vi "Calculate Center.vi"(8 "Type of Assembly Tray":i32, 9 "Syringe Coordinates":dbl[](array[numeric]), 10 "Relative Coordinates":dbl[][](array[numeric]), 11 "Fiducial Measurements":dbl[][](array[numeric])) -> (3 "XYZTheta Centers":dbl[][](array[numeric]))   [LabVIEW 2019, in "Assembly Tray.lvclass"]
uses:
  Assembly Tray.lvclass
  <vilib>/Analysis/coordinate.llb/2D Cartesian Coordinate Rotation (Scalar).vi
  <vilib>/Analysis/NI_AALPro.lvlib
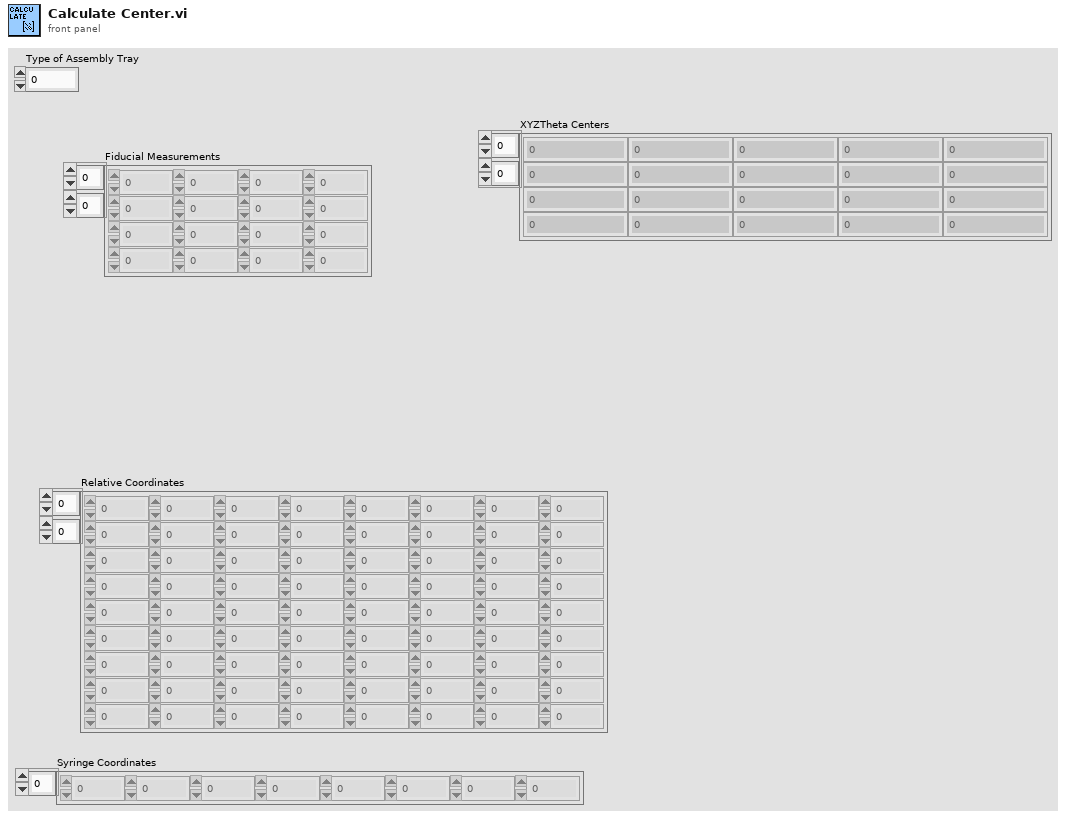
[diagram p1: front panel]
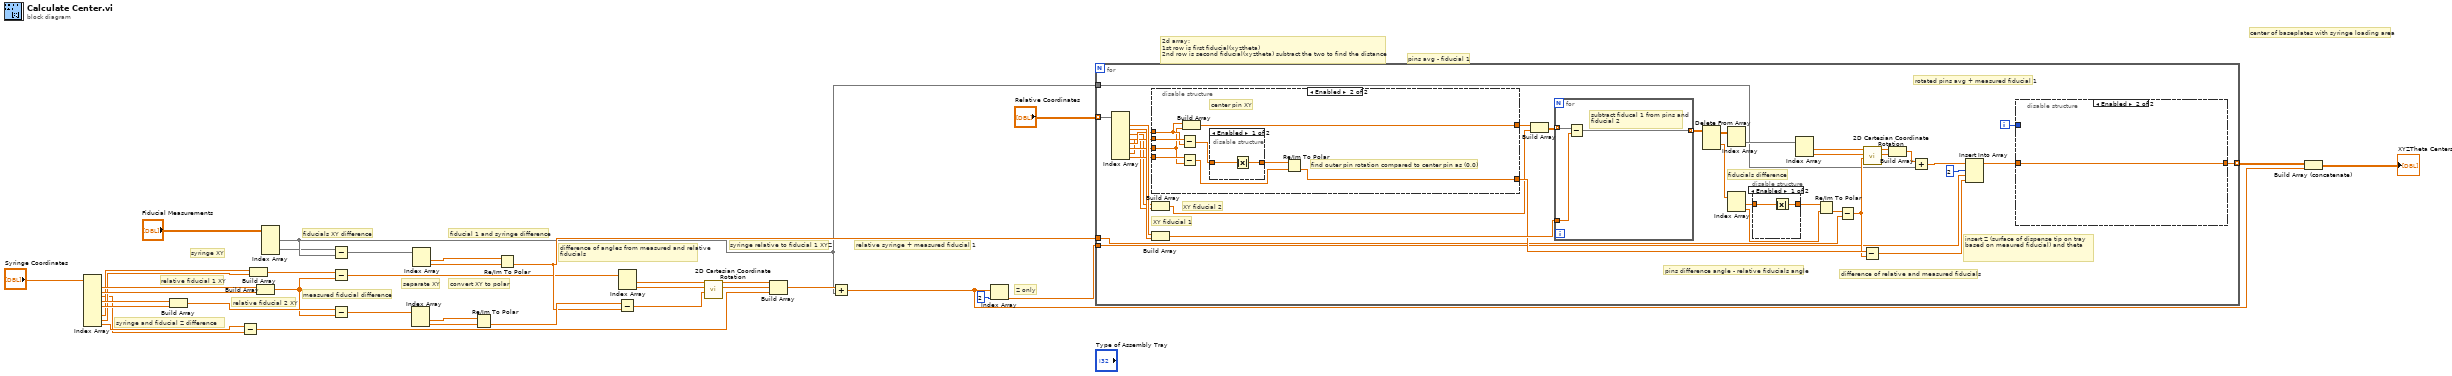
[diagram p0: block diagram]
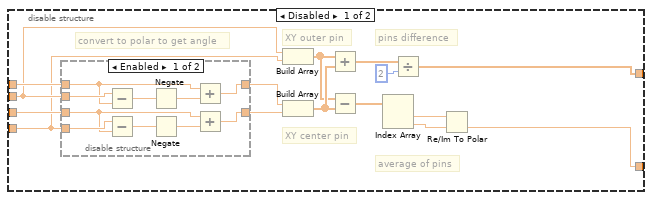
[diagram p3: hidden frame]
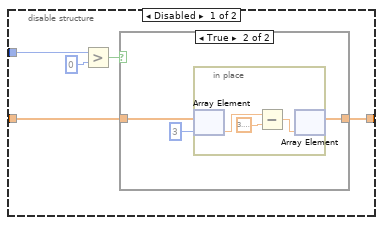
[diagram p6: hidden frame]
diagram:
  # "center of baseplates with syringe loading area"
  # "relative fiducial 2 XY"
  # "relative fiducial 1 XY"
  # "syringe XY"
  # "pins avg - fiducial 1"
  # "Z only"
  # "relative syringe + measured fiducial 1"
  # "syringe relative to fiducial 1 XYZ"
  # "difference of angles from measured and relative fiducials"
  # "separate XY"
  # "convert XY to polar"
  # "measured fiducial difference"
  # "fiducial 1 and syringe difference"
  # "syringe and fiducial Z difference"
  # "fiducials XY difference"
  # "2d array:\n1st row is first fiducial(xyztheta)\n2nd row is second fiducial(xyztheta) subtract the two to find the distance"
  n1 = Index Array(array="Syringe Coordinates") -> (element #1=w32:dbl, element #2=w31:dbl, element #3=w13:dbl, element #4=w29:dbl, element #5=w28:dbl, element #7=w16:dbl, element #8=w15:dbl, element #9=w14:dbl)  [unwired: 9 in, 1 out]
  n2 = Build Array(w29, w28) -> (w30:dbl[])
  n3 = Subtract(x=w14, y=w13) -> (x-y=w4:dbl)
  n4 = Build Array(w16, w15) -> (w21:dbl[])
  n5 = Build Array(w32, w31) -> (w20:dbl[])
  n6 = Index Array(array="Fiducial Measurements") -> (element #1=w2:dbl[], element #2=w1:dbl[])  [unwired: 4 in]
  n7 = Subtract(x=w1, y=w2) -> (x-y=w7:dbl[])
  n8 = Subtract(x=w21, y=w20) -> (x-y=w19:dbl[])
  n9 = Subtract(x=w30, y=w20) -> (x-y=w27:dbl[])
  n10 = Index Array(array=w27) -> (element #1=w26:dbl, element #2=w25:dbl)  [unwired: 2 in]
  n11 = Index Array(array=w7) -> (element #1=w35:dbl, element #2=w36:dbl)  [unwired: 2 in]
  n12 = Re/Im To Polar(2:w25, 3:w26) -> (0:w24:dbl)  [unwired: 1 out]
  n13 = Re/Im To Polar(2:w36, 3:w35) -> (0:w23:dbl)  [unwired: 1 out]
  n14 = Subtract(x=w24, y=w23) -> (x-y=w22:dbl)
  n15 = Index Array(array=w19) -> (element #1=w18:dbl, element #2=w17:dbl)  [unwired: 2 in]
  n16 = call-poly <vilib>:"2D Cartesian Coordinate Rotation.vi"("theta"=w22, "y"=w17, "x"=w18) -> ("y out"=w11:dbl, "x out"=w12:dbl)  [unwired: 6 in, 1 out]
  n17 = Build Array(w12, w11, w4) -> (w8:dbl[])
  n18 = Add(x=w8, y=w2) -> (x+y=w3:dbl[])
  n19 = Index Array(array=w3, index=2) -> (element=w5:dbl)
  n20 = for {
    tunnel: "Relative Coordinates" -> [w54] mode=indexing
    tunnel: [w45] -> w10 mode=indexing
    tunnel: w2 -> [w53]
    tunnel: w23 -> [w52]
    tunnel: w5 -> [w51]
    i -> [w44]
    # "insert Z (surface of dispense tip on tray based on meaured fiducial) and theta"
    # "pins difference angle - relative fiducials angle"
    # "rotated pins avg + measured fiducial 1"
    # "difference of relative and measured fiducials"
    # "fiducials difference"
    # "XY fiducial 2"
    # "XY fiducial 1"
    n21 = Index Array(array=w54) -> (element #1=w74:dbl, element #2=w73:dbl, element #3=w43:dbl, element #4=w42:dbl, element #5=w49:dbl, element #6=w50:dbl, element #7=w48:dbl, element #8=w47:dbl)  [unwired: 8 in]
    n22 = disable-structure shown="Enabled" {
      disable-tunnel: [w90 w105] -> w58
      disable-tunnel: [w84 w109] -> w56
      disable-tunnel: w50 -> [w81 w106]
      disable-tunnel: w49 -> [w80 w107]
      disable-tunnel: w48 -> [w79 w110]
      disable-tunnel: w47 -> [w78 w108]
      frame Disabled {
        # "convert to polar to get angle"
        # "pins difference"
        # "average of pins"
        # "XY outer pin"
        # "XY center pin"
        n23 = disable-structure shown="Enabled" {
          disable-tunnel: w78 -> [w102 _]
          disable-tunnel: w79 -> [w101 _]
          disable-tunnel: w81 -> [w98 w104]
          disable-tunnel: w80 -> [w95 w103]
          disable-tunnel: [w94 w104] -> w82
          disable-tunnel: [w93 w103] -> w83
          frame Enabled {
            n24 = Subtract(x=w101, y=w95) -> (x-y=w99:dbl)
            n25 = Subtract(x=w102, y=w98) -> (x-y=w100:dbl)
            n26 = Negate(x=w99) -> (-x=w96:dbl)
            n27 = Negate(x=w100) -> (-x=w97:dbl)
            n28 = Add(x=w95, y=w96) -> (x+y=w93:dbl)
            n29 = Add(x=w98, y=w97) -> (x+y=w94:dbl)
          }
          frame Disabled {
          }
        }
        n30 = Build Array(w79, w78) -> (w88:dbl[])
        n31 = Build Array(w83, w82) -> (w89:dbl[])
        n32 = Add(x=w88, y=w89) -> (x+y=w91:dbl[])
        n33 = Subtract(x=w88, y=w89) -> (x-y=w87:dbl[])
        n34 = Index Array(array=w87) -> (element #1=w86:dbl, element #2=w85:dbl)  [unwired: 2 in]
        n35 = Divide(x=w91, y=2) -> (x/y=w90:dbl[])
        n36 = Re/Im To Polar(2:w85, 3:w86) -> (0:w84:dbl)  [unwired: 1 out]
      }
      frame Enabled {
        # "find outer pin rotation compared to center pin as (0,0)"
        # "center pin XY"
        n37 = Subtract(x=w110, y=w107) -> (x-y=w112:dbl)
        n38 = Subtract(x=w108, y=w106) -> (x-y=w113:dbl)
        n39 = Build Array(w107, w106) -> (w105:dbl[])
        n40 = disable-structure shown="Enabled" {
          disable-tunnel: w112 -> [w115 w116]
          disable-tunnel: [w114 w116] -> w111
          frame Enabled {
            n41 = Absolute Value(x=w115) -> (abs(x)=w114:dbl)
          }
          frame Disabled {
          }
        }
        n42 = Re/Im To Polar(2:w113, 3:w111) -> (0:w109:dbl)  [unwired: 1 out]
      }
    }
    n43 = Build Array(w43, w42) -> (w41:dbl[])
    n44 = Build Array(w74, w73) -> (w71:dbl[])
    n45 = Build Array(w58, w41) -> (w72:dbl[][])
    n46 = for {
      tunnel: w72 -> [w132] mode=indexing
      tunnel: w71 -> [w131]
      tunnel: [w130] -> w70 mode=indexing
      # "subtract fiducal 1 from pins and fiducial 2"
      n47 = Subtract(x=w132, y=w131) -> (x-y=w130:dbl[])
    }
    n48 = Delete From Array(array=w70) -> (deleted portion=w69:dbl[], array with subset deleted=w67:dbl[][])  [unwired: 3 in]
    n49 = Index Array(array=w67) -> (element=w66:dbl[])  [unwired: 2 in]
    n50 = Index Array(array=w69) -> (element #1=w40:dbl, element #2=w68:dbl)  [unwired: 2 in]
    n51 = disable-structure shown="Enabled" {
      disable-tunnel: w40 -> [w76 w77]
      disable-tunnel: [w75 w77] -> w39
      frame Enabled {
        n52 = Absolute Value(x=w76) -> (abs(x)=w75:dbl)
      }
      frame Disabled {
      }
    }
    n53 = Index Array(array=w66) -> (element #1=w65:dbl, element #2=w64:dbl)  [unwired: 2 in]
    n54 = Re/Im To Polar(2:w68, 3:w39) -> (0:w57:dbl)  [unwired: 1 out]
    n55 = Subtract(x=w57, y=w52) -> (x-y=w55:dbl)
    n56 = Subtract(x=w56, y=w55) -> (x-y=w38:dbl)
    n57 = call-poly <vilib>:"2D Cartesian Coordinate Rotation.vi"("theta"=w55, "y"=w64, "x"=w65) -> ("y out"=w61:dbl, "x out"=w62:dbl)  [unwired: 6 in, 1 out]
    n58 = Build Array(w62, w61) -> (w63:dbl[])
    n59 = Add(x=w63, y=w53) -> (x+y=w60:dbl[])
    n60 = Insert Into Array(array=w60, index=2, new element #1=w51, new element #2=w38) -> (w46:dbl[])
    n61 = disable-structure shown="Enabled" {
      disable-tunnel: w46 -> [w121 w129]
      disable-tunnel: [w120 w129] -> w45
      disable-tunnel: w44 -> [w117 _]
      frame Disabled {
        n62 = Greater?(x=w117, y=0) -> (0:w118:bool)
        n63 = case shown="True" w118 {
          tunnel: w121 -> [w122 w124]
          tunnel: [w122 w123] -> w120
          frame False {
          }
          frame True {
            n64 = in-place {
              n65 = in-place-array #1(w124, 3) -> (w128:dbl)
              n66 = Subtract(x=w128, y=3.141592653589793) -> (x-y=w127:dbl)
              n67 = in-place-array #1(w127) -> (w123:dbl[])  [unwired: 1 out]
            }
          }
        }
      }
      frame Enabled {
      }
    }
  }
  n68 = Build Array (concatenate)(w10, w3) -> (→"XYZTheta Centers":dbl[][])
